vi "putBallAsObstacleInPotentialField.vi"(6 "ArrayOfObstacles in":T1[](array[typedef]), 9 "multiplier":dbl, 10 "influence radius":dbl, 11 "Ball in":refnum<class "Ball.lvclass">) -> (3 "ArrayOfObstacles out":T1[](array[typedef]))   [LabVIEW 2020, in "Robot.lvclass"]
uses:
  Robot.lvclass
  obstacle.ctl
  Ball_class/Ball.lvclass
  C:/RoboIME/SSL_AI/Object_class/Object.lvclass
  Object_class/Object.lvclass/Object.ctl
  Object_class/Read x.vi
  Object_class/Read y.vi
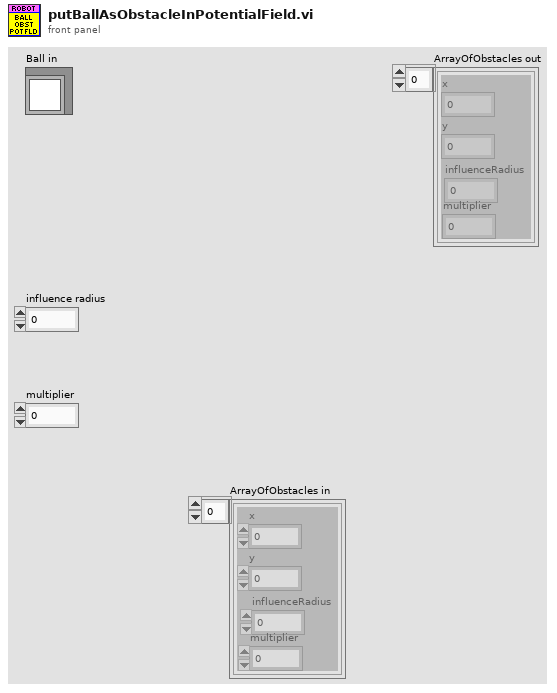
[diagram p1: front panel]
types:
  T1 = typedef "obstacle.ctl" = cluster{"x":dbl, "y":dbl, "influenceRadius":dbl, "multiplier":dbl}
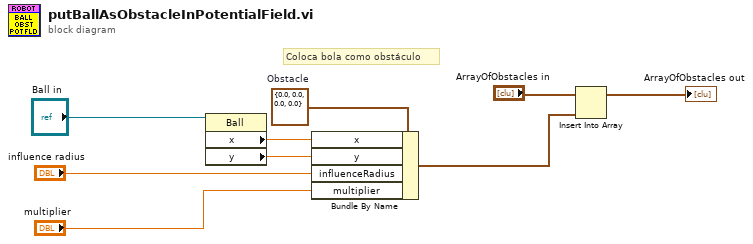
[diagram p0: block diagram]
diagram:
  w2 = T1 {"x"=0.0, "y"=0.0, "influenceRadius"=0.0, "multiplier"=0.0}  # Obstacle
  # "Coloca bola como obstáculo"
  n1 = property class="Ball"(reference="Ball in") -> ("x"=w3:dbl, "y"=w4:dbl)  [unwired: 1 in, 2 out]
  n2 = Bundle By Name(cluster=w2, "x"=w3, "y"=w4, "influenceRadius"="influence radius", "multiplier"="multiplier") -> (w6:T1)
  n3 = Insert Into Array(array="ArrayOfObstacles in", new element=w6) -> (→"ArrayOfObstacles out":T1[])  [unwired: 1 in]
